vi "WFGCheckConfigValid.vi"(0 "object in":refnum<class "AD2_WFG_SDK.lvclass">, 2 "Ch":T1={"idxChannel"=0, "Settings out of range"=FALSE, "Carrier"={"Frequency (Hz)"=1000.0, "Amplitude (V)"=1.0, "Offset(V)"=0.0, "Symmetry(%) "=50.0, "Phase(Deg)"=0.0, "Function"=1, "Enable"=FALSE}, "Trigger"={"secRun(0=Cont)"=0.0, "secWait"=0.0, "cRepeat(0=inf)"=0, "Repeat Trigger"=FALSE, "TrigrSrc"=enum."trigrsrcNone"}, "FM Mod"={"Frequency (Hz)"=1000.0, "Amplitude (%)"=1.0, "Offset(V)"=0.0, "Symmetry(%) "=50.0, "Phase(Deg)"=0.0, "Function 2"=1, "Enable"=FALSE}} {"FM Mod"."Function 2" items=["DC"=0, "Sine"=1, "Square"=2, "Triangle"=3, "RampUp"=4, "RampDown"=5, "Noise"=6, "Pulse"=7, "Custom"=30]; "Carrier"."Function" items=["DC"=0, "Sine"=1, "Square"=2, "Triangle"=3, "RampUp"=4, "RampDown"=5, "Noise"=6, "Pulse"=7, "Custom"=30]}, 5 "error in (no error)":errorcluster) -> (14 "object out":refnum<class "AD2_WFG_SDK.lvclass">, 15 "Settings Coerced!":bool, 16 "Ch Out":T1={"idxChannel"=0, "Settings out of range"=FALSE, "Carrier"={"Frequency (Hz)"=1000.0, "Amplitude (V)"=1.0, "Offset(V)"=0.0, "Symmetry(%) "=50.0, "Phase(Deg)"=0.0, "Function"=1, "Enable"=TRUE}, "Trigger"={"secRun(0=Cont)"=0.0, "secWait"=0.0, "cRepeat(0=inf)"=0, "Repeat Trigger"=FALSE, "TrigrSrc"=enum."trigrsrcNone"}, "FM Mod"={"Frequency (Hz)"=1000.0, "Amplitude (%)"=1.0, "Offset(V)"=0.0, "Symmetry(%) "=50.0, "Phase(Deg)"=0.0, "Function 2"=1, "Enable"=FALSE}} {"FM Mod"."Function 2" items=["DC"=0, "Sine"=1, "Square"=2, "Triangle"=3, "RampUp"=4, "RampDown"=5, "Noise"=6, "Pulse"=7, "Custom"=30]; "Carrier"."Function" items=["DC"=0, "Sine"=1, "Square"=2, "Triangle"=3, "RampUp"=4, "RampDown"=5, "Noise"=6, "Pulse"=7, "Custom"=30]}, 19 "error out":errorcluster)   [LabVIEW 2021, in "AD2_WFG_SDK.lvclass"]
uses:
  AD2_WFG_SDK.lvclass
  WFGCh.ctl
  AD2TriggerSources.ctl
  AD2_WFG_SDK.lvclass/AD2_WFG_SDK.ctl
  Olasdwf/Olasdwf.lvlib
  AD2_SDK_class/AD2_SDK.lvclass
panel:
  out "coerced(x)":dbl
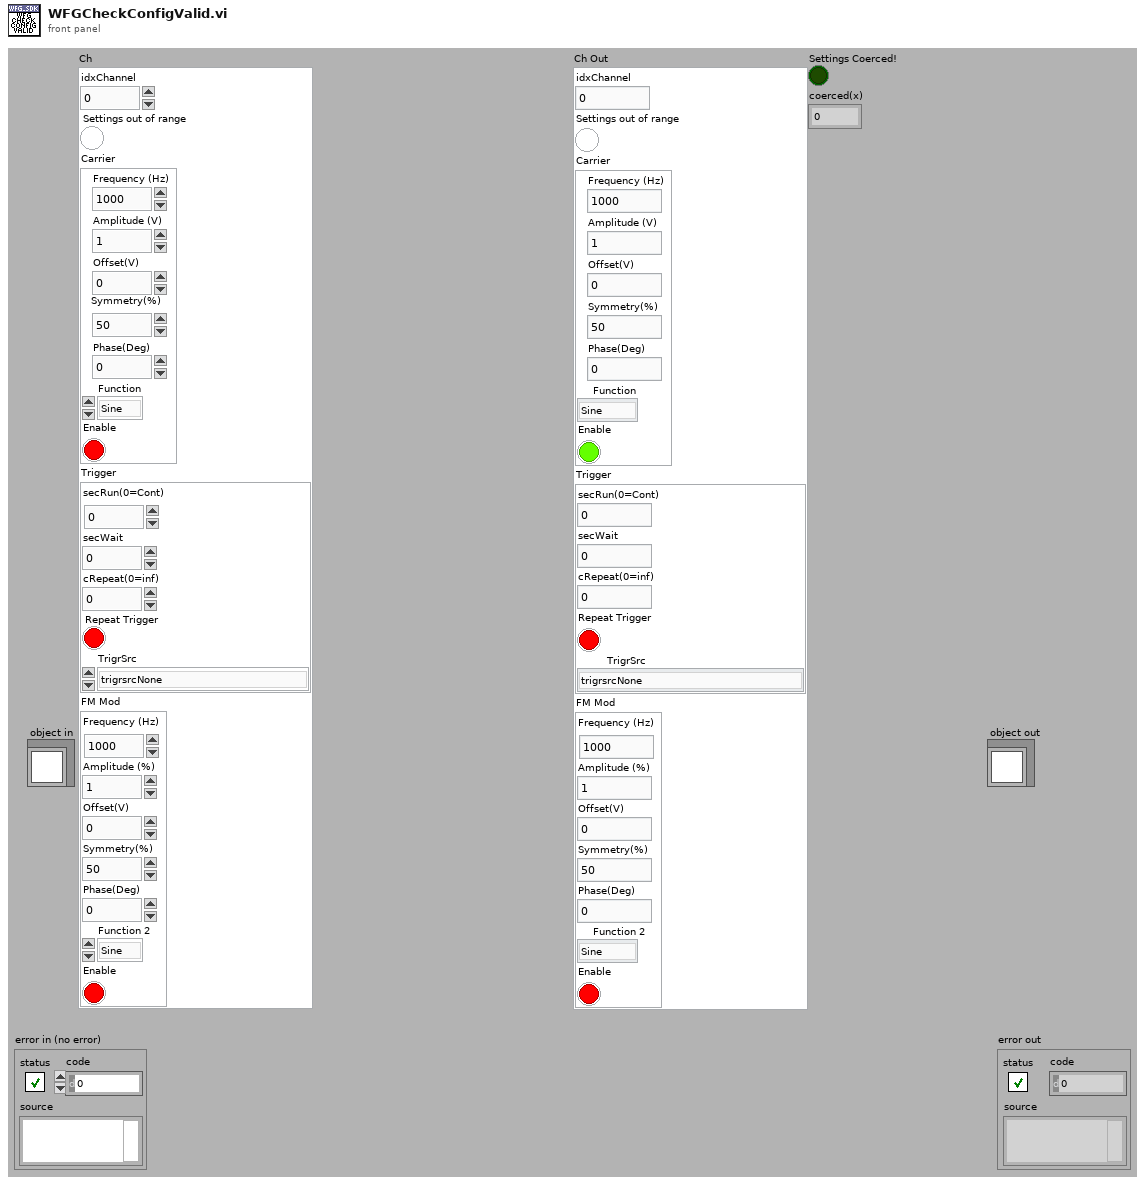
[diagram p1: front panel]
types:
  T1 = typedef "AD2_WFG_SDK.lvclass/WFGCh.ctl" = cluster{"idxChannel":i32, "Settings out of range":bool, "Carrier":cluster{"Frequency (Hz)":dbl, "Amplitude (V)":dbl, "Offset(V)":dbl, "Symmetry(%) ":dbl, "Phase(Deg)":dbl, "Function":u16, "Enable":bool}, "Trigger":cluster{"secRun(0=Cont)":dbl, "secWait":dbl, "cRepeat(0=inf)":i32, "Repeat Trigger":bool, "TrigrSrc":T2}, "FM Mod":cluster{"Frequency (Hz)":dbl, "Amplitude (%)":dbl, "Offset(V)":dbl, "Symmetry(%) ":dbl, "Phase(Deg)":dbl, "Function 2":u16, "Enable":bool}}
  T2 = typedef "AD2_SDK.lvclass/AD2TriggerSources.ctl" = enum8{"trigrsrcNone", "trigsrcPC", "trigsrcDetectorAnalogIn", "trigsrcDetectorDigitalIn", "trigsrcAnalogIn", "trigsrcDigitalIn", "trigsrcDigitalOut", "trigsrcAnalogOut1", "trigsrcAnalogOut2", "trigsrcAnalogOut3", "trigsrcAnalogOut4", "trigsrcExternal1", "trigsrcExternal2", "trigsrcExternal3", "trigsrcExternal4", ""}
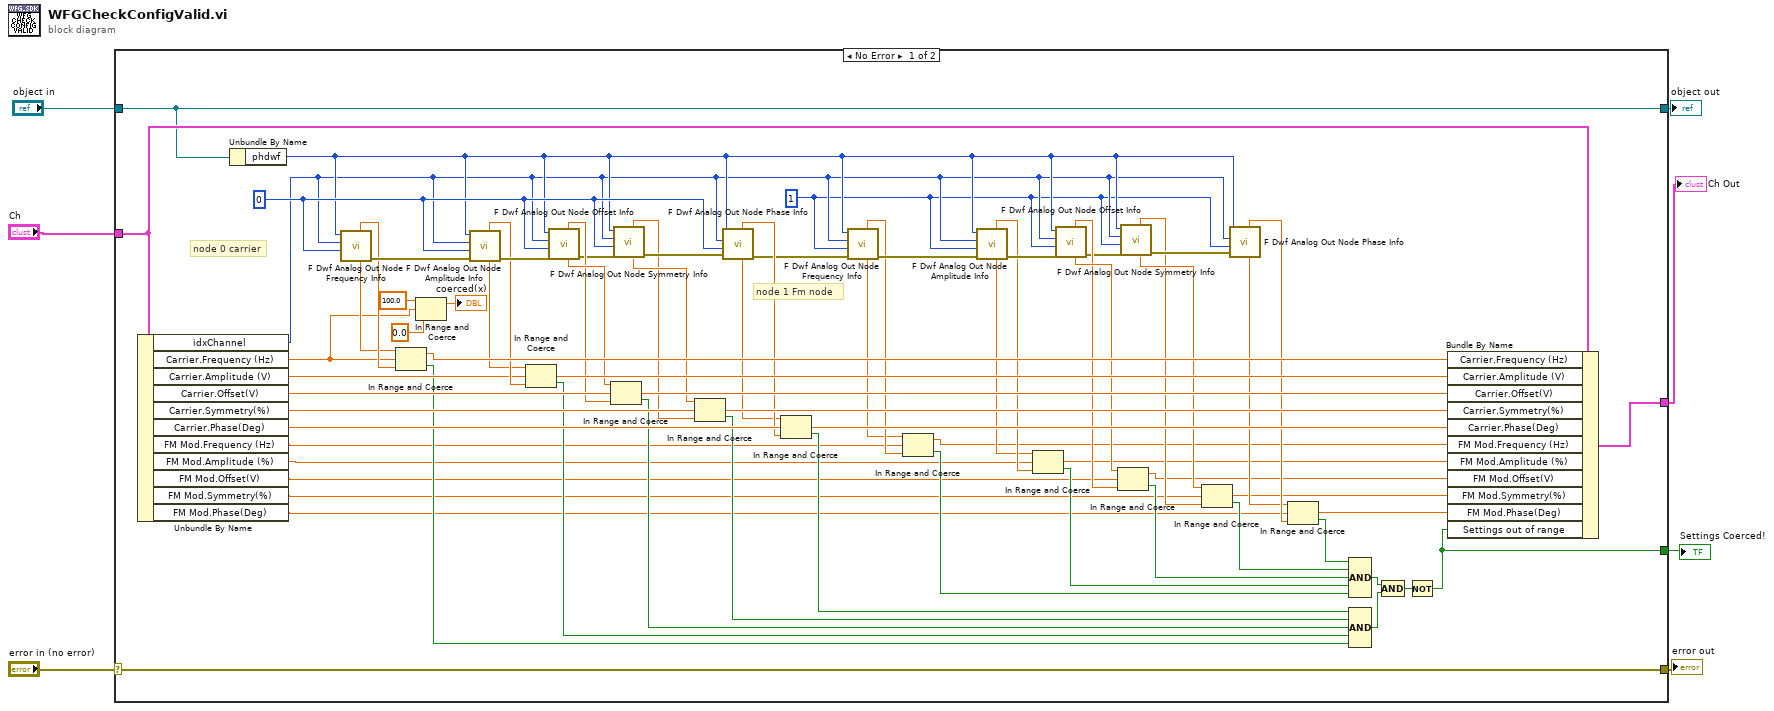
[diagram p0: block diagram]
diagram:
  n1 = case shown="No Error" "error in (no error)" {
    selector: "error in (no error)" -> [w81 w83]
    tunnel: [w81 w83] -> w6
    tunnel: [w49 w82] -> w4
    tunnel: "object in" -> [w49 w82]
    tunnel: "Ch" -> [w76 _]
    tunnel: [w55 _] -> w2
    tunnel: [w8 _] -> w1
    frame No Error {
      w26 = 1 ("node")
      w56 = 0 ("node")
      # "node 1 Fm node"
      # "node 0 carrier"
      n2 = Unbundle By Name(w76) -> ("idxChannel"=w27:i32, "Carrier.Frequency (Hz)"=w11:dbl, "Carrier.Amplitude (V)"=w72:dbl, "Carrier.Offset(V)"=w70:dbl, "Carrier.Symmetry(%)"=w66:dbl, "Carrier.Phase(Deg)"=w63:dbl, "FM Mod.Frequency (Hz)"=w20:dbl, "FM Mod.Amplitude (%)"=w19:dbl, "FM Mod.Offset(V)"=w18:dbl, "FM Mod.Symmetry(%)"=w17:dbl, "FM Mod.Phase(Deg)"=w16:dbl)
      n3 = Unbundle By Name(w49) -> ("phdwf"=w28:i32)
      n4 = call "F Dwf Analog Out Node Frequency Info.vi"("node"=w56, "idxChannel"=w27, "hdwf"=w28) -> ("error out"=w80:errorcluster, "phzMax out"=w77:dbl, "phzMin out"=w78:dbl)  [unwired: 5 in, 1 out]
      n5 = In Range and Coerce(upper limit=w77, x=w11, lower limit=w78) -> (coerced(x)=w75:dbl, In Range?=w50:bool)
      n6 = In Range and Coerce(upper limit=100.0, x=w11, lower limit=0.0) -> (coerced(x)=→"coerced(x)":dbl)  [unwired: 1 out]
      n7 = call "F Dwf Analog Out Node Amplitude Info.vi"("error in (no error)"=w80, "node"=w56, "idxChannel"=w27, "hdwf"=w28) -> ("error out"=w79:errorcluster, "pMax out"=w73:dbl, "pMin out"=w74:dbl)  [unwired: 4 in, 1 out]
      n8 = In Range and Coerce(upper limit=w73, x=w72, lower limit=w74) -> (coerced(x)=w71:dbl, In Range?=w51:bool)
      n9 = call "F Dwf Analog Out Node Offset Info.vi"("error in (no error)"=w79, "node"=w56, "idxChannel"=w27, "hdwf"=w28) -> ("error out"=w60:errorcluster, "pMax out"=w68:dbl, "pMin out"=w67:dbl)  [unwired: 4 in, 1 out]
      n10 = In Range and Coerce(upper limit=w68, x=w70, lower limit=w67) -> (coerced(x)=w69:dbl, In Range?=w52:bool)
      n11 = call "F Dwf Analog Out Node Symmetry Info.vi"("error in (no error)"=w60, "node"=w56, "idxChannel"=w27, "hdwf"=w28) -> ("error out"=w59:errorcluster, "ppercentageMax out"=w58:dbl, "ppercentageMin out"=w57:dbl)  [unwired: 4 in, 1 out]
      n12 = In Range and Coerce(upper limit=w58, x=w66, lower limit=w57) -> (coerced(x)=w65:dbl, In Range?=w53:bool)
      n13 = call "F Dwf Analog Out Node Phase Info.vi"("error in (no error)"=w59, "node"=w56, "idxChannel"=w27, "hdwf"=w28) -> ("error out"=w29:errorcluster, "pdegreeMax out"=w61:dbl, "pdegreeMin out"=w62:dbl)  [unwired: 4 in, 1 out]
      n14 = In Range and Coerce(upper limit=w61, x=w63, lower limit=w62) -> (coerced(x)=w64:dbl, In Range?=w54:bool)
      n15 = call "F Dwf Analog Out Node Frequency Info.vi"("error in (no error)"=w29, "node"=w26, "idxChannel"=w27, "hdwf"=w28) -> ("error out"=w48:errorcluster, "phzMax out"=w45:dbl, "phzMin out"=w46:dbl)  [unwired: 4 in, 1 out]
      n16 = In Range and Coerce(upper limit=w45, x=w20, lower limit=w46) -> (coerced(x)=w25:dbl, In Range?=w30:bool)
      n17 = call "F Dwf Analog Out Node Amplitude Info.vi"("error in (no error)"=w48, "node"=w26, "idxChannel"=w27, "hdwf"=w28) -> ("error out"=w47:errorcluster, "pMax out"=w43:dbl, "pMin out"=w44:dbl)  [unwired: 4 in, 1 out]
      n18 = In Range and Coerce(upper limit=w43, x=w19, lower limit=w44) -> (coerced(x)=w21:dbl, In Range?=w31:bool)
      n19 = call "F Dwf Analog Out Node Offset Info.vi"("error in (no error)"=w47, "node"=w26, "idxChannel"=w27, "hdwf"=w28) -> ("error out"=w38:errorcluster, "pMax out"=w42:dbl, "pMin out"=w41:dbl)  [unwired: 4 in, 1 out]
      n20 = In Range and Coerce(upper limit=w42, x=w18, lower limit=w41) -> (coerced(x)=w22:dbl, In Range?=w32:bool)
      n21 = call "F Dwf Analog Out Node Symmetry Info.vi"("error in (no error)"=w38, "node"=w26, "idxChannel"=w27, "hdwf"=w28) -> ("error out"=w37:errorcluster, "ppercentageMax out"=w36:dbl, "ppercentageMin out"=w35:dbl)  [unwired: 4 in, 1 out]
      n22 = In Range and Coerce(upper limit=w36, x=w17, lower limit=w35) -> (coerced(x)=w23:dbl, In Range?=w33:bool)
      n23 = call "F Dwf Analog Out Node Phase Info.vi"("error in (no error)"=w37, "node"=w26, "idxChannel"=w27, "hdwf"=w28) -> ("pdegreeMax out"=w39:dbl, "pdegreeMin out"=w40:dbl)  [unwired: 4 in, 2 out]
      n24 = In Range and Coerce(upper limit=w39, x=w16, lower limit=w40) -> (coerced(x)=w24:dbl, In Range?=w34:bool)
      n25 = Compound Arithmetic op=AND(w34, w33, w32, w31, w30) -> (w15:bool)
      n26 = Compound Arithmetic op=AND(w54, w53, w52, w51, w50) -> (w14:bool)
      n27 = Compound Arithmetic op=AND(w15, w14) -> (w9:bool)
      n28 = Not(x=w9) -> (.not. x?=w8:bool)
      n29 = Bundle By Name(cluster=w76, "Carrier.Frequency (Hz)"=w75, "Carrier.Amplitude (V)"=w71, "Carrier.Offset(V)"=w69, "Carrier.Symmetry(%)"=w65, "Carrier.Phase(Deg)"=w64, "FM Mod.Frequency (Hz)"=w25, "FM Mod.Amplitude (%)"=w21, "FM Mod.Offset(V)"=w22, "FM Mod.Symmetry(%)"=w23, "FM Mod.Phase(Deg)"=w24, "Settings out of range"=w8) -> (w55:T1)
    }
    frame Error {
    }
  }
  "error out" <- w6
  "object out" <- w4
  "Ch Out" <- w2
  "Settings Coerced!" <- w1
